vi "Number Decomposition.VI"(0 "number string":string, 1 "error in (no error)":errorcluster) -> (2 "number":string, 3 "rest":string, 4 "error out":errorcluster)   [LabVIEW 2018, in "NI_Gmath.lvlib"]
uses:
  NI_Gmath.lvlib
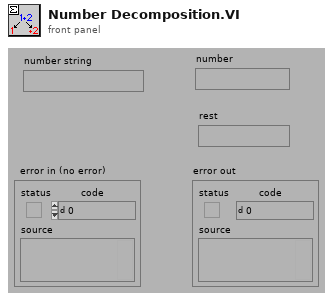
[diagram p1: front panel]
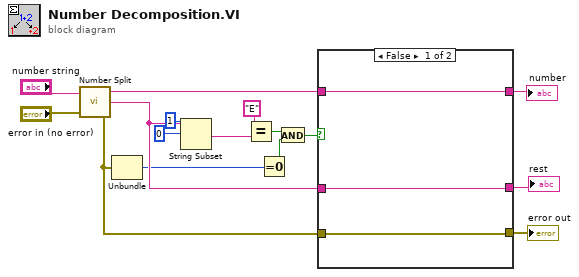
[diagram p0: block diagram]
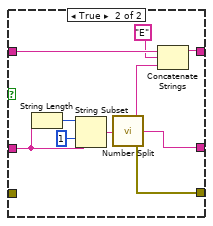
[diagram p2: hidden frame]
diagram:
  n1 = call "Number Split.VI"("number string"="number string", "error in (no error)"="error in (no error)") -> ("number"=w8:string, "rest"=w12:string, "error out"=w1:errorcluster)
  n2 = Unbundle(w1) -> ("code"=w4:i32)  [unwired: 2 out]
  n3 = String Subset(string=w12, offset (0)=0, length (rest)=1) -> (substring=w5:string)
  n4 = Equal?(x="E", y=w5) -> (x = y?=w10:bool)
  n5 = Equal To 0?(x=w4) -> (x = 0?=w9:bool)
  n6 = And(x=w10, y=w9) -> (x .and. y?=w6:bool)
  n7 = case shown="False" w6 {
    tunnel: w12 -> [w19 w29]
    tunnel: [w19 w25] -> w11
    tunnel: w8 -> [w18 w24]
    tunnel: [w18 w23] -> w7
    tunnel: [w17 w20] -> w2
    tunnel: w1 -> [w17 _]
    frame False {
    }
    frame True {
      n8 = String Length(string=w29) -> (length=w28:i32)
      n9 = String Subset(string=w29, offset (0)=1, length (rest)=w28) -> (substring=w26:string)
      n10 = call "Number Split.VI"("number string"=w26) -> ("number"=w21:string, "rest"=w25:string, "error out"=w20:errorcluster)  [unwired: 1 in]
      n11 = Concatenate Strings(w24, "E", w21) -> (w23:string)
    }
  }
  "number" <- w7
  "rest" <- w11
  "error out" <- w2
